vi "NAttackersPositionPenalty.vi"(0 "N atacantes":u32[](array[numeric]), 1 "Total de n \natacantes":i32) -> (7 "Posição dos não atacantes\ndurante o penalte":dbl[][](array[numeric]))   [LabVIEW 2016]
panel:
  in  "Array  in":dbl[][](array[numeric])=[[99999.0, 99999.0], [99999.0, 99999.0], [99999.0, 99999.0], [99999.0, 99999.0], [99999.0, 99999.0], [99999.0, 99999.0], [99999.0, 99999.0]]
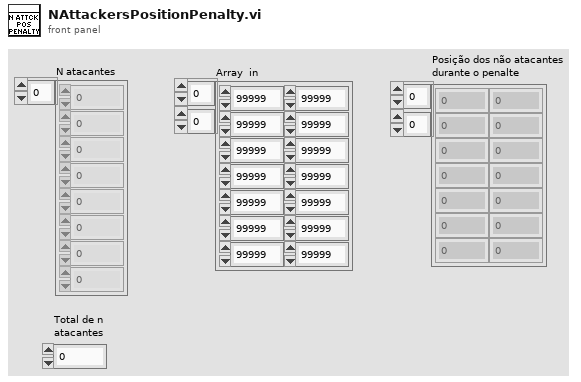
[diagram p1: front panel]
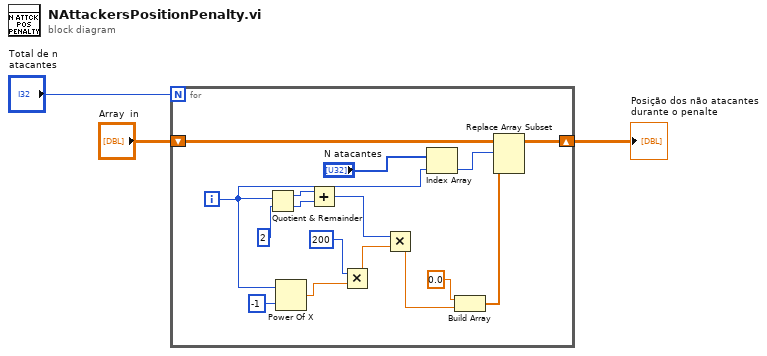
[diagram p0: block diagram]
diagram:
  n1 = for {
    N: "Total de n \natacantes" -> [_]
    shift-right: [w6] -> w3
    shift-left: "Array  in" -> [w7]
    i -> [w4]
    n2 = Quotient & Remainder(x=w4, y=2) -> (x-y*floor(x/y)=w16:i32, floor(x/y)=w15:i32)
    n3 = Power Of X(1:-1 ("x"), 2:w4) -> (0:w18:dbl)
    n4 = Add(x=w16, y=w15) -> (x+y=w14:i32)
    n5 = Multiply(x=200, y=w18) -> (x*y=w13:dbl)
    n6 = Multiply(x=w14, y=w13) -> (x*y=w12:dbl)
    n7 = Index Array(array="N atacantes", index=w4) -> (element=w9:u32)
    n8 = Build Array(0.0 ("element"), w12) -> (w5:dbl[])
    n9 = Replace Array Subset(array=w7, new element=w5, index (row)=w9) -> (w6:dbl[][])  [unwired: 1 in]
  }
  "Posição dos não atacantes\ndurante o penalte" <- w3
